vi "panel_hardware_resource_checkin.vi"(7 "Self":bool=TRUE, 8 "error in (no error)":errorcluster, 9 "panel_number":T1, 10 "hardware.lvclass":refnum<class "hardware.lvclass">, 11 "panel in":refnum<class "panel.lvclass">) -> (0 "error out":errorcluster, 3 "panel out":refnum<class "panel.lvclass">)   [LabVIEW 2015, in "panel.lvclass"]
uses:
  panel.lvclass
  Hardware Class/hardware/hardware.lvclass
  front_panel_class/hardware_caller_queue_numbers.ctl
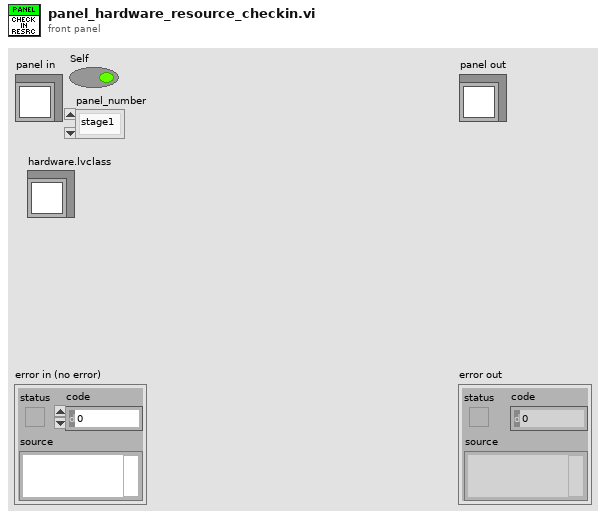
[diagram p1: front panel]
types:
  T1 = typedef "hardware_caller_queue_numbers.ctl" = enum16{"stage1", "stage2", "experiment", "detector"}
  T2 = typedef "hardware_seqs.ctl" = refnum<queue>[]
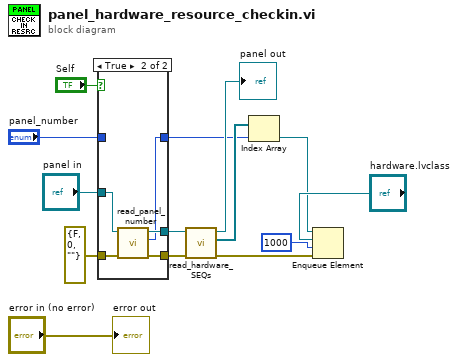
[diagram p0: block diagram]
diagram:
  n1 = case shown="True" "Self" {
    tunnel: errorcluster {"status"=FALSE, "code"=0, "source"=""} ("error in (no error)") -> [w15 w22]
    tunnel: [w15 w21] -> w9
    tunnel: "panel in" -> [w16 w20]
    tunnel: [w16 w19] -> w8
    tunnel: [w17 w18] -> w6
    tunnel: "panel_number" -> [w17 _]
    frame False {
    }
    frame True {
      n2 = call "read_panel_number.vi"("error in (no error)"=w22, "panel in"=w20) -> ("error out"=w21:errorcluster, "panel_number"=w18:T1, "panel out"=w19:refnum<class "panel.lvclass">)  [unwired: 7 in]
    }
  }
  n3 = call "read_hardware_SEQs.vi"("error in (no error)"=w9, "panel in"=w8) -> ("error out"=w4:errorcluster, "hardware_SEQs"=w7:T2, "panel out"=→"panel out":refnum<class "panel.lvclass">)  [unwired: 7 in]
  n4 = Index Array(array=w7, index=w6) -> (element=w5:refnum<queue>)
  n5 = Enqueue Element(queue=w5, element="hardware.lvclass", timeout in ms (-1)=1000, error in (no error)=w4) -> ()  [unwired: 3 out]
  "error out" <- "error in (no error)"
